vi "ao_waveform_sync.vi"() -> ()   [LabVIEW 2020]
uses:
  <vilib>/measure/NI_MABase.lvlib
panel:
  in  "Offset":dbl
  in  "signal type":T1(ring) caption="Signal Type"
  out "error out":errorcluster caption="错误输出"
  in  "Frequency":dbl=1000.0 format="%#.6g"
  in  "Amplitude":dbl=5.0 format="%.3f"
  out "波形图":waveform(dbl)(graph)
  in  "AoCycle":u32
  in  "SamplePeriod (ns)":u32=10000
  in  "DevIndex":i32
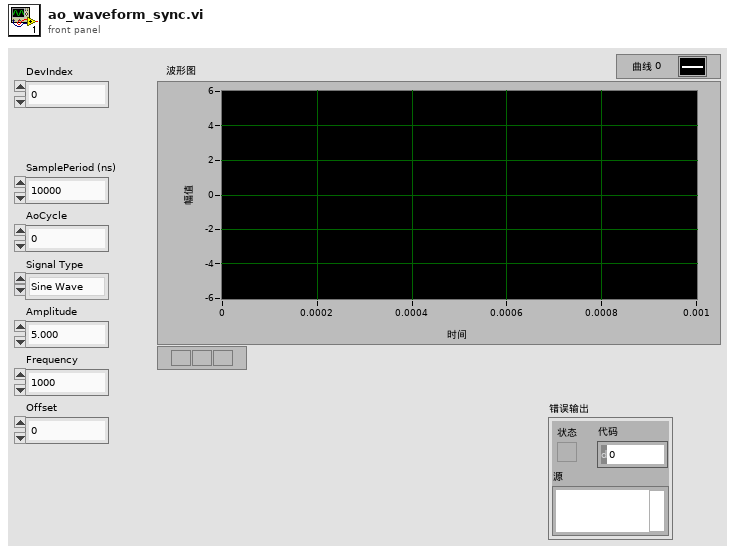
[diagram p1: front panel]
types:
  T1 = enum16{"Sine Wave", "Triangle Wave", "Square Wave", "Sawtooth Wave"}
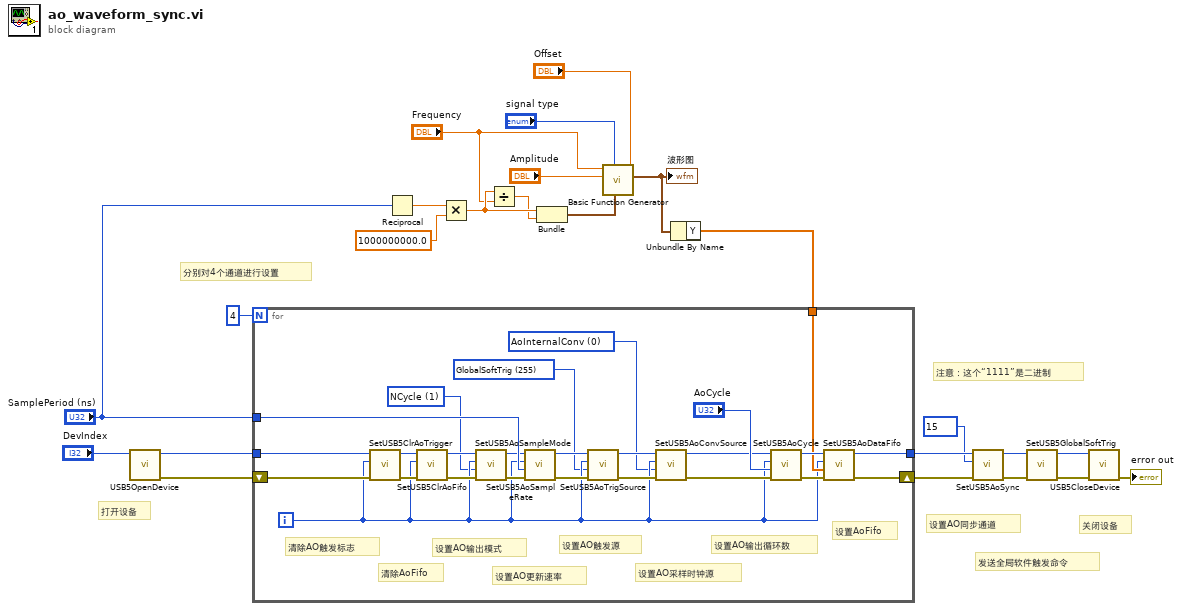
[diagram p0: block diagram]
diagram:
  # "关闭设备"
  # "发送全局软件触发命令"
  # "注意：这个“1111”是二进制"
  # "设置AO同步通道"
  # "分别对4个通道进行设置"
  # "打开设备"
  n1 = call "USB5OpenDevice.vi"("DevIndex"="DevIndex") -> ("error out"=w22:errorcluster, "DevIndex Out"=w21:i32)  [unwired: 9 in]
  n2 = Reciprocal(x="SamplePeriod (ns)") -> (1/x=w20:dbl)
  n3 = Multiply(x=w20, y=1000000000.0) -> (x*y=w17:dbl)
  n4 = Divide(x=w17, y="Frequency") -> (x/y=w16:dbl)
  n5 = Bundle(w17, w16) -> (w19:cluster{dbl, dbl})  [unwired: 1 in]
  n6 = call <vilib>:"Basic Function Generator.vi"("offset"="Offset", "sampling info"=w19, "signal type"="signal type", "amplitude"="Amplitude", "frequency"="Frequency") -> ("signal out"=w13:waveform(dbl))  [unwired: 4 in, 2 out]
  "波形图" <- w13
  n7 = Unbundle By Name(w13) -> ("Y"=w12:dbl[])
  n8 = for {
    N: 4 -> [_]
    tunnel: "SamplePeriod (ns)" -> [w47]
    tunnel: w12 -> [w41]
    shift-right: [w48] -> w4
    shift-left: w22 -> [w46]
    tunnel: w21 -> [w45]
    tunnel: [w49] -> w6
    i -> [w28]
    w25 = u8 0 items=["AoInternalConv", "ConvIn", "AiConv", "DiConv", "DoConv", "Ao0Conv", "Ao1Conv", "Ao2Conv", "Ao3Conv"] ("AoConvSource")
    w26 = u8 255 items=["AoSoftTrig"=0, "ExtTrigIn"=1, "Din0RisingEdge"=2, "Din1RisingEdge"=3, "Din2RisingEdge"=4, "Din3RisingEdge"=5, "WithAiTrig"=6, "WithDiTrig"=7, "WithDoTrig"=8, "WithAo0Trig"=9, "WithAo1Trig"=10, "WithAo2Trig"=11, "WithAo3Trig"=12, "GlobalSoftTrig"=255] ("AoTrigSource")
    w27 = u8 1 items=["PcBufferedInfinite", "NCycle"] ("SampleMode")
    # "设置AoFifo"
    # "设置AO输出循环数"
    # "设置AO采样时钟源"
    # "设置AO触发源"
    # "设置AO更新速率"
    # "设置AO输出模式"
    # "清除AoFifo"
    # "清除AO触发标志"
    n9 = call "SetUSB5ClrAoTrigger.vi"("错误输入（无错误）"=w46, "Chan"=w28, "DevIndex"=w45) -> ("错误输出"=w40:errorcluster, "DevIndex Out"=w39:i32)  [unwired: 7 in]
    n10 = call "SetUSB5ClrAoFifo.vi"("错误输入（无错误）"=w40, "Chan"=w28, "DevIndex"=w39) -> ("错误输出"=w37:errorcluster, "DevIndex Out"=w38:i32)  [unwired: 7 in]
    n11 = call "SetUSB5AoSampleMode.vi"("错误输入（无错误）"=w37, "SampleMode"=w27, "Chan"=w28, "DevIndex"=w38) -> ("错误输出"=w36:errorcluster, "DevIndex Out"=w35:i32)  [unwired: 6 in]
    n12 = call "SetUSB5AoSampleRate.vi"("错误输入（无错误）"=w36, "SamplePeriod(ns)"=w47, "Chan"=w28, "DevIndex"=w35) -> ("错误输出"=w33:errorcluster, "DevIndex Out"=w34:i32)  [unwired: 6 in]
    n13 = call "SetUSB5AoTrigSource.vi"("错误输入（无错误）"=w33, "AoTrigSource"=w26, "Chan"=w28, "DevIndex"=w34) -> ("错误输出"=w31:errorcluster, "DevIndex Out"=w32:i32)  [unwired: 6 in]
    n14 = call "SetUSB5AoConvSource.vi"("错误输入（无错误）"=w31, "AoConvSource"=w25, "Chan"=w28, "DevIndex"=w32) -> ("错误输出"=w29:errorcluster, "DevIndex Out"=w30:i32)  [unwired: 6 in]
    n15 = call "SetUSB5AoCycle.vi"("错误输入（无错误）"=w29, "AoCycle"="AoCycle", "Chan"=w28, "DevIndex"=w30) -> ("错误输出"=w43:errorcluster, "DevIndex Out"=w42:i32)  [unwired: 6 in]
    n16 = call "SetUSB5AoDataFifo.vi"("错误输入（无错误）"=w43, "Voltage"=w41, "Chan"=w28, "DevIndex"=w42) -> ("错误输出"=w48:errorcluster, "DevIndex Out"=w49:i32)  [unwired: 6 in]
  }
  n17 = call "SetUSB5AoSync.vi"("错误输入（无错误）"=w4, "Chans"=u8 15, "DevIndex"=w6) -> ("错误输出"=w3:errorcluster, "DevIndex Out"=w5:i32)  [unwired: 7 in]
  n18 = call "SetUSB5GlobalSoftTrig.vi"("错误输入（无错误）"=w3, "DevIndex"=w5) -> ("错误输出"=w7:errorcluster, "DevIndex Out"=w8:i32)  [unwired: 8 in]
  n19 = call "USB5CloseDevice.vi"("错误输入（无错误）"=w7, "DevIndex"=w8) -> ("error out"=→"error out":errorcluster)  [unwired: 8 in, 1 out]
